vi "Get Next Transfer Size (private).vi"(0 "data in":T1, 5 "error in (no error)":errorcluster) -> (14 "data out":T1, 15 "elements to transfer":u32, 19 "error out":errorcluster)   [LabVIEW 2021, in "Disk Streaming.lvclass"]
doc: "Returns the size of the next block to transfer.\n\nInputs:\n\n<B>data in</B>: Disk streaming data input.\n\nOutputs:\n\n<B>data out</B>: Disk streaming data output.\n\n<B>elements to transfer</B>: The number of elements the next block should transfer. If this output is zero, then the streaming is complete."
uses:
  Disk Streaming.lvclass
  Data.ctl
  Public/IO mode.ctl
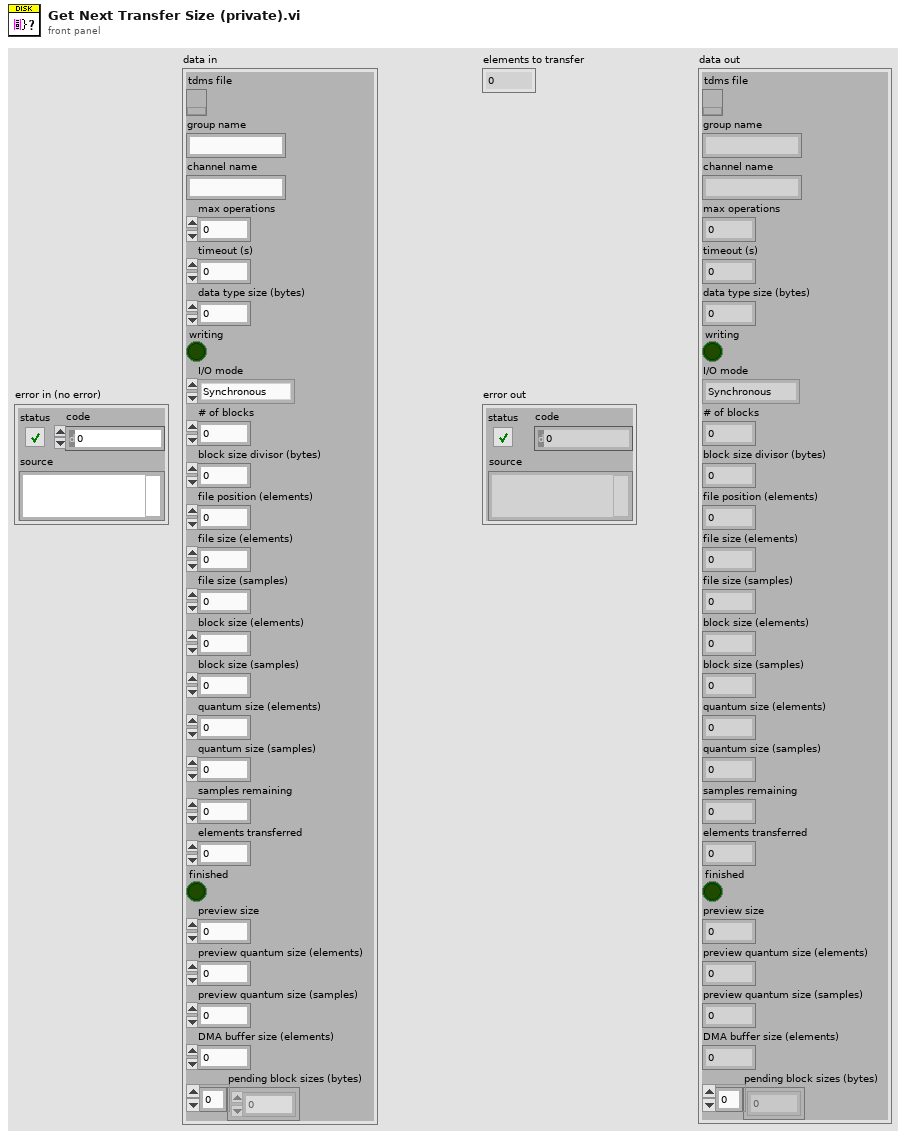
[diagram p1: front panel]
types:
  T1 = typedef "Disk Streaming.lvclass/Data.ctl" = cluster{"tdms file":refnum<k34>, "group name":string, "channel name":string, "max operations":u32, "timeout (s)":dbl, "data type size (bytes)":u64, "writing":bool, "I/O mode":T2, "# of blocks":u32, "block size divisor (bytes)":u32, "file position (elements)":u64, "file size (elements)":i64, "file size (samples)":i64, "block size (elements)":u64, "block size (samples)":u64, "quantum size (elements)":u64, "quantum size (samples)":u64, "samples remaining":i64, "elements transferred":u64, "finished":bool, "preview size":i32, "preview quantum size (elements)":u64, "preview quantum size (samples)":u64, "DMA buffer size (elements)":u32, "pending block sizes (bytes)":u64[]}
  T2 = typedef "Disk Streaming.lvclass/IO mode.ctl" = enum16{"Synchronous", "Asynchronous", "Data Reference"}
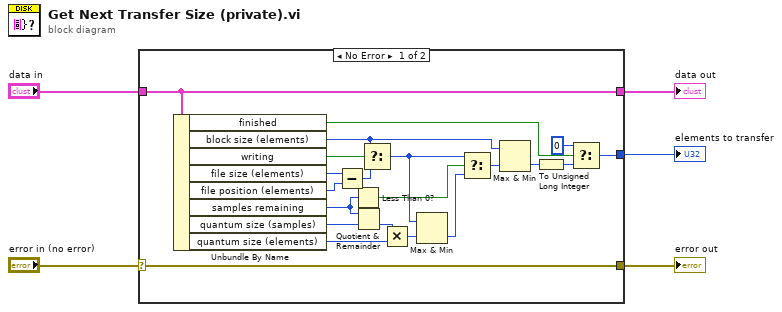
[diagram p0: block diagram]
diagram:
  n1 = case shown="No Error" "error in (no error)" {
    selector: "error in (no error)" -> [w7 w28]
    tunnel: [w7 w28] -> w4
    tunnel: "data in" -> [w6 w27]
    tunnel: [w26 _] -> w3
    tunnel: [w6 w27] -> w1
    frame No Error {
      n2 = Unbundle By Name(w6) -> ("finished"=w9:bool, "block size (elements)"=w12:u64, "writing"=w23:bool, "file size (elements)"=w25:i64, "file position (elements)"=w24:u64, "samples remaining"=w15:i64, "quantum size (samples)"=w21:u64, "quantum size (elements)"=w20:u64)
      n3 = Subtract(x=w25, y=w24) -> (x-y=w22:u64)
      n4 = Less Than 0?(x=w15) -> (x < 0?=w14:bool)
      n5 = Quotient & Remainder(x=w15, y=w21) -> (floor(x/y)=w19:u64)  [unwired: 1 out]
      n6 = Select(t=w12, s=w23, f=w22) -> (s? t:f=w17:u64)
      n7 = Multiply(x=w19, y=w20) -> (x*y=w18:u64)
      n8 = Max & Min(x=w17, y=w18) -> (min(x,y)=w16:u64)  [unwired: 1 out]
      n9 = Select(t=w17, s=w14, f=w16) -> (s? t:f=w13:u64)
      n10 = Max & Min(x=w12, y=w13) -> (min(x,y)=w11:u64)  [unwired: 1 out]
      n11 = To Unsigned Long Integer(number=w11) -> (unsigned 32bit integer=w10:u32)
      n12 = Select(t=u32 0, s=w9, f=w10) -> (s? t:f=w26:u32)
    }
    frame Error {
    }
  }
  "error out" <- w4
  "elements to transfer" <- w3
  "data out" <- w1
